vi "BallPosition.vi"(8 "balls":T1[](array[typedef]), 9 "IA State":T2={"our_robots"=[], "enemy_robots"=[], "balls"=[], "geometry"={"field_length"=0, "field_width"=0, "goal_width"=0, "goal_depth"=0, "center_circle_radius"=0, "defense_width"=0, "defense_depth"=0, "free_kick_from_defense_dist"=0, "penalty_spot_from_field_line_dist"=0, "penalty_line_from_spot_dist"=0, "half_moon_depth"=0, "half_moon_width"=0}, "IA Judge"={"stage"="", "command"="", "our_goalie_id"=0.0, "enemy_goalie_id"=0.0, "command enum"=enum."Halt", "Time"=enum."Azul"}, "Received Timestamp"=timestamp(0 s since 1904-01-01), "Events"={"Touch"=FALSE, "id touch"=0.0, "Ball out of \nVision"=FALSE, "Ball inside \nGoalie area"=FALSE, "Robot not responding"=FALSE, "Robots responding status"=[1.0, 1.0, 1.0, 1.0, 1.0, 1.0], "Enemy Ball \nPossession"=FALSE, "Id ini Possession"=0.0, "Ball Possesion"=FALSE, "Id Possesion"=0.0, "Ball at\nour goal side"=FALSE, "Ball at\ntouchline"=FALSE, "Ball at\nenemy goal side"=FALSE}}, 11 "Robot in":T3) -> (3 "Robot out":T3)   [LabVIEW 2018]
uses:
  Core/AI Robot.ctl
  Functions Enum.ctl
  AttackerStates.ctl
  Path Planning/RRT/PathDests.ctl
  Path Planning/RRT/PathDest.ctl
  Core/AI Input.ctl
  Core/AI Ball.ctl
  Core/Field Size.ctl
  Core/AI Judge.ctl
  Command Enum.ctl
  Util/Events/Events.ctl
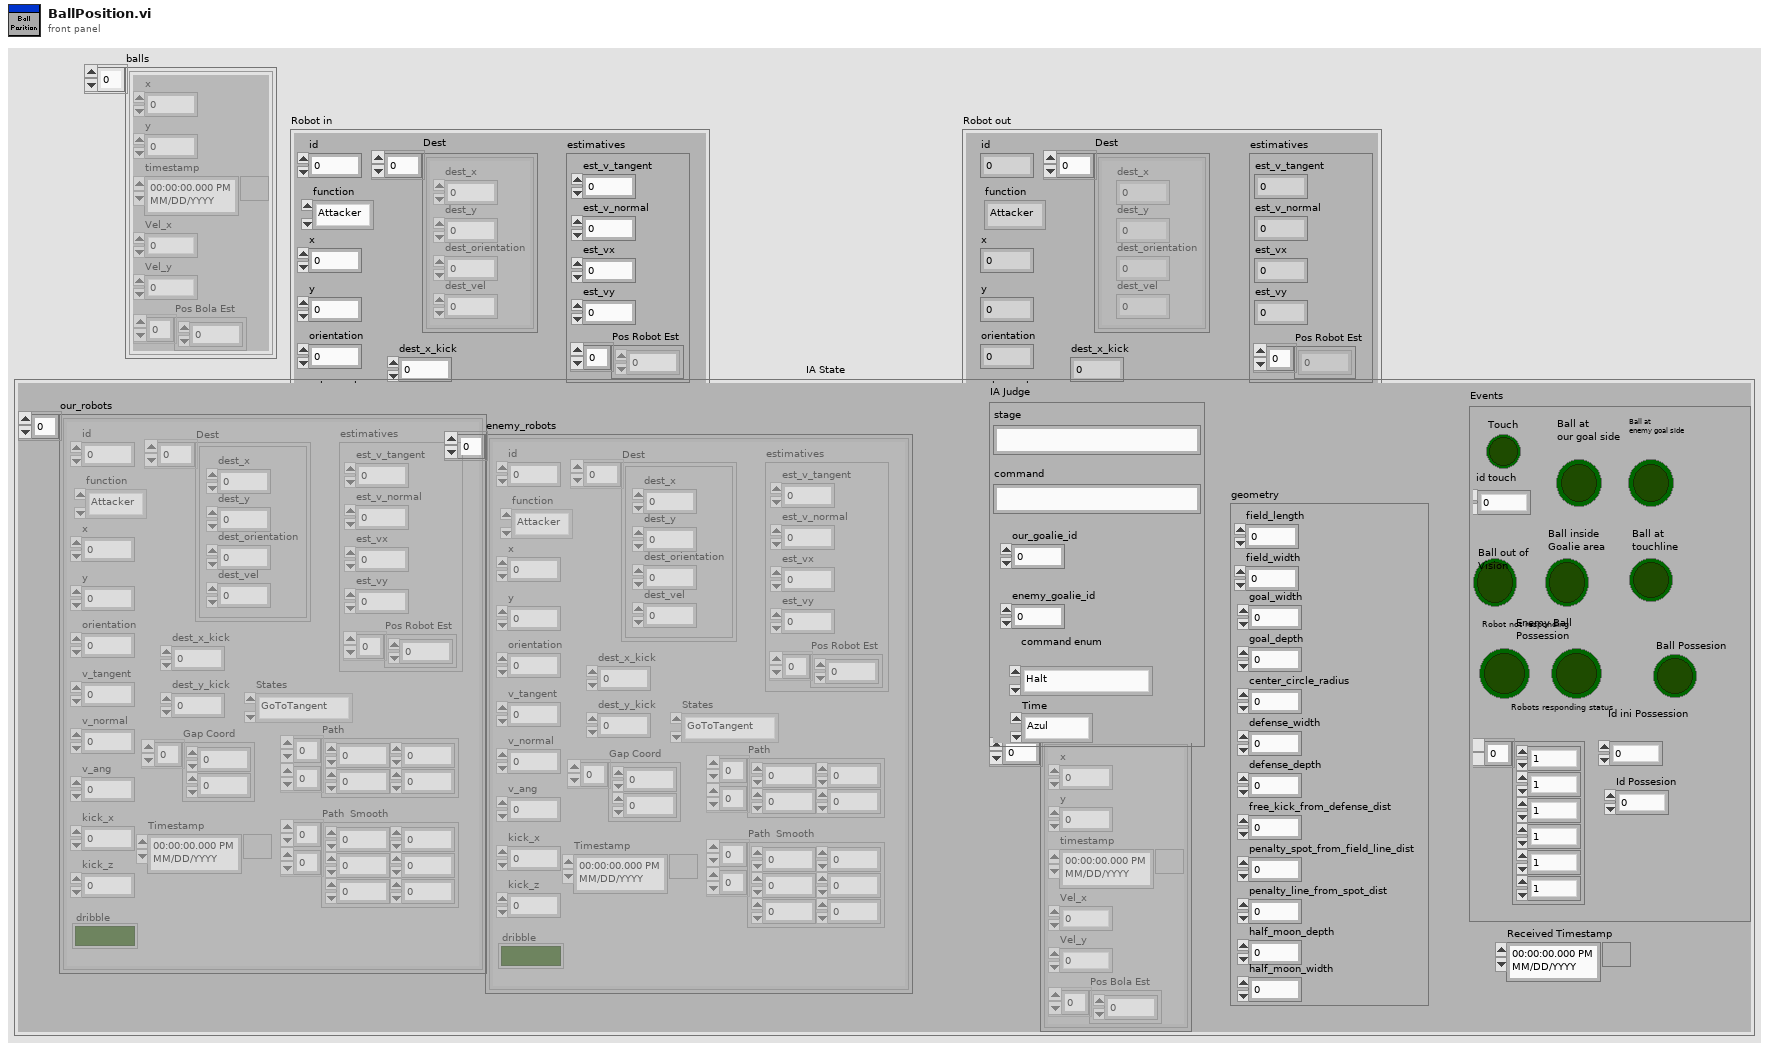
[diagram p1: front panel]
types:
  T1 = typedef "AI Ball.ctl" = cluster{"x":dbl, "y":dbl, "timestamp":timestamp, "Vel_x":dbl, "Vel_y":dbl, "Pos Bola Est":dbl[]}
  T2 = typedef "AI Input.ctl" = cluster{"our_robots":T3[], "enemy_robots":T3[], "balls":T1[], "geometry":T8, "IA Judge":T9, "Received Timestamp":timestamp, "Events":T11}
  T3 = typedef "AI Robot.ctl" = cluster{"id":u32, "function":T4, "x":dbl, "y":dbl, "orientation":dbl, "v_tangent":dbl, "v_normal":dbl, "v_ang":dbl, "kick_x":dbl, "kick_z":dbl, "dribble":bool, "Timestamp":timestamp, "estimatives":cluster{"est_v_tangent":dbl, "est_v_normal":dbl, "est_vx":dbl, "est_vy":dbl, "Pos Robot Est":dbl[]}, "dest_x_kick":dbl, "dest_y_kick":dbl, "Gap Coord":dbl[], "States":T5, "Path ":dbl[][], "Path  Smooth":dbl[][], "Dest":T6}
  T4 = typedef "Functions Enum.ctl" = enum16{"Attacker", "Goalie", "Defender", "Striker", "Goto 0", "Dummy", "Kicker", "ZigZag"}
  T5 = typedef "AttackerStates.ctl" = enum16{"Pass", "GoToTangent", "BallGetting", "GoToKick", "Rotate anti-clockwise", "Rotate Clockwise", ""}
  T6 = typedef "PathDests.ctl" = T7[]
  T7 = typedef "PathDest.ctl" = cluster{"dest_x":dbl, "dest_y":dbl, "dest_orientation":dbl, "dest_vel":dbl}
  T8 = typedef "Field Size.ctl" = cluster{"field_length":u32, "field_width":u32, "goal_width":u32, "goal_depth":u32, "center_circle_radius":u32, "defense_width":u32, "defense_depth":u32, "free_kick_from_defense_dist":u32, "penalty_spot_from_field_line_dist":u32, "penalty_line_from_spot_dist":u32, "half_moon_depth":u32, "half_moon_width":u32}
  T9 = typedef "AI Judge.ctl" = cluster{"stage":string, "command":string, "our_goalie_id":dbl, "enemy_goalie_id":dbl, "command enum":T10, "Time":enum16{"Azul", "Amarelo"}}
  T10 = typedef "Command Enum.ctl" = enum16{"Halt", "Stop", "Force Start", "PKA Normal Start", "Prepare Kickoff Ally", "PKE Normal Start", "Prepare Kickoff Enemy", "Prepare Penalty Ally", "PPA Normal Start", "Prepare Penalty Enemy", "PPE Normal Start", "Ball Placement Enemy Up", "Ball Placement Enemy Down", "Ball Placement Ally Up", "Ball Placement Ally Mid", "Ball Placement Ally Down", "Indirect Free Enemy", "Indirect Free Ally", "Timeout Enemy", "Timeout Ally", "Goal Enemy", "Goal Ally", "Normal Half Time", "Extra Time Break", "Extra Half Time", "None", "Post Game"}
  T11 = typedef "Events.ctl" = cluster{"Touch":bool, "id touch":dbl, "Ball out of \nVision":bool, "Ball inside \nGoalie area":bool, "Robot not responding":bool, "Robots responding status":dbl[], "Enemy Ball \nPossession":bool, "Id ini Possession":dbl, "Ball Possesion":bool, "Id Possesion":dbl, "Ball at\nour goal side":bool, "Ball at\ntouchline":bool, "Ball at\nenemy goal side":bool}
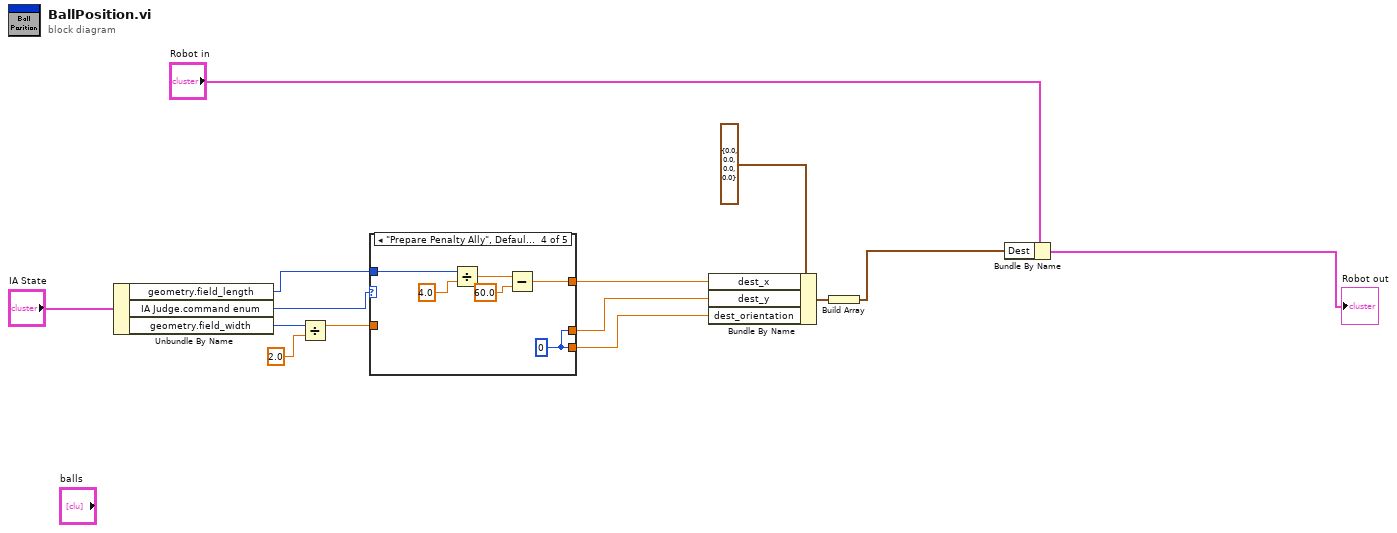
[diagram p0: block diagram]
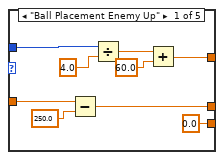
[diagram p2: hidden frame]
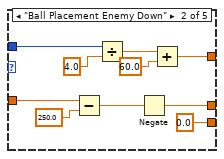
[diagram p3: hidden frame]
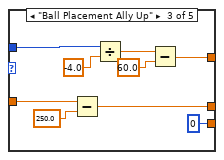
[diagram p4: hidden frame]
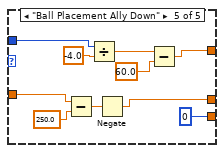
[diagram p5: hidden frame]
diagram:
  n1 = Unbundle By Name("IA State") -> ("geometry.field_length"=w4:u32, "IA Judge.command enum"=w8:T10, "geometry.field_width"=w7:u32)
  n2 = Divide(x=w7, y=2.0) -> (x/y=w6:dbl)
  n3 = case shown="\"Prepare Penalty Ally\", Default" w8 {
    tunnel: w6 -> [w16 w26 w42 _ w52]
    tunnel: [w17 w24 w40 w43 w50] -> w2
    tunnel: [0.0 0.0 0 w43 0] -> w1
    tunnel: w4 -> [w19 w29 w37 w45 w54]
    tunnel: [w18 w28 w35 w44 w53] -> w3
    frame "Ball Placement Enemy Up" {
      n4 = Subtract(x=w16, y=250.0) -> (x-y=w17:dbl)
      n5 = Divide(x=w19, y=4.0) -> (x/y=w21:dbl)
      n6 = Add(x=w21, y=60.0) -> (x+y=w18:dbl)
    }
    frame "Ball Placement Enemy Down" {
      n7 = Subtract(x=w26, y=250.0) -> (x-y=w25:dbl)
      n8 = Divide(x=w29, y=4.0) -> (x/y=w33:dbl)
      n9 = Negate(x=w25) -> (-x=w24:dbl)
      n10 = Add(x=w33, y=60.0) -> (x+y=w28:dbl)
    }
    frame "Ball Placement Ally Up" {
      n11 = Subtract(x=w42, y=250.0) -> (x-y=w40:dbl)
      n12 = Divide(x=w37, y=-4.0) -> (x/y=w36:dbl)
      n13 = Subtract(x=w36, y=60.0) -> (x-y=w35:dbl)
    }
    frame "Prepare Penalty Ally", Default {
      w43 = 0
      n14 = Divide(x=w45, y=4.0) -> (x/y=w47:dbl)
      n15 = Subtract(x=w47, y=60.0) -> (x-y=w44:dbl)
    }
    frame "Ball Placement Ally Down" {
      n16 = Subtract(x=w52, y=250.0) -> (x-y=w51:dbl)
      n17 = Divide(x=w54, y=-4.0) -> (x/y=w56:dbl)
      n18 = Negate(x=w51) -> (-x=w50:dbl)
      n19 = Subtract(x=w56, y=60.0) -> (x-y=w53:dbl)
    }
  }
  n20 = Bundle By Name(cluster=T7 {"dest_x"=0.0, "dest_y"=0.0, "dest_orientation"=0.0, "dest_vel"=0.0} ("element"), "dest_x"=w3, "dest_y"=w2, "dest_orientation"=w1) -> (w13:T7)
  n21 = Build Array(w13) -> (w14:T7[])
  n22 = Bundle By Name(cluster="Robot in", "Dest"=w14) -> (→"Robot out":T3)
